vi "Create_filter_points_Sub.vi"(1 "Numeric Value?":bool[](array[boolean]), 4 "No of filter options":i32=100, 5 "Precision":string, 6 "Tolerance":dbl=1.0 format="%.2f", 7 "Bin Matches in":bool[][](array[boolean]), 8 "Numeric Array":dbl[](array[numeric]) format="%.2f", 9 "Bin Names In":string[](array[string]), 10 "String Array":string[](array[string])) -> (2 "Bin Matches":bool[][](array[boolean]), 3 "Bin Names":string[](array[string]))   [LabVIEW 2021]
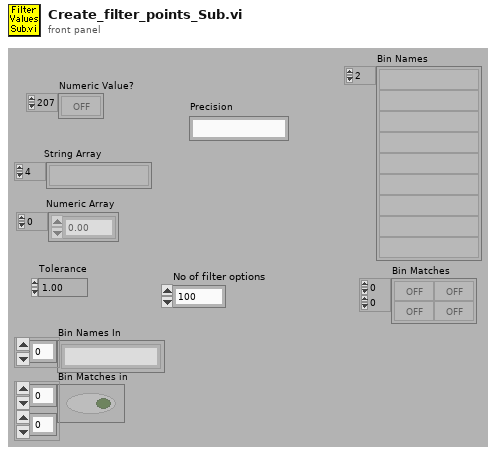
[diagram p1: front panel]
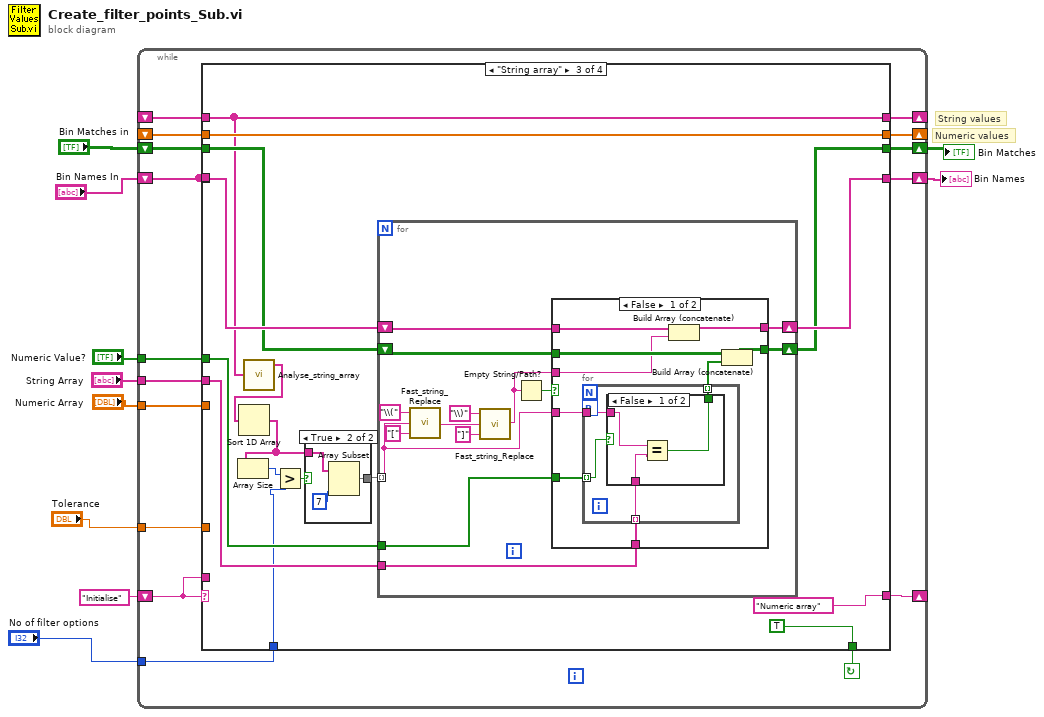
[diagram p0: block diagram]
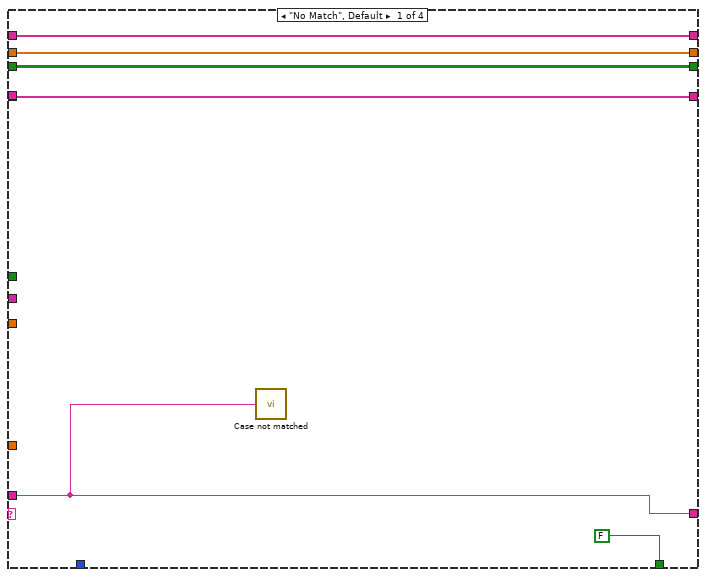
[diagram p2: hidden frame]
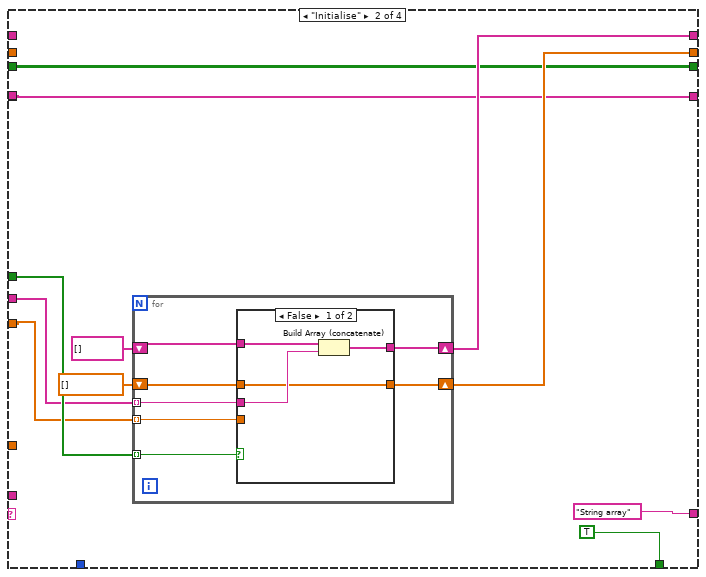
[diagram p3: hidden frame]
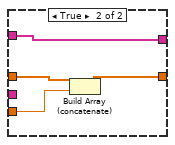
[diagram p4: hidden frame]
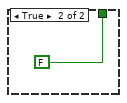
[diagram p6: hidden frame]
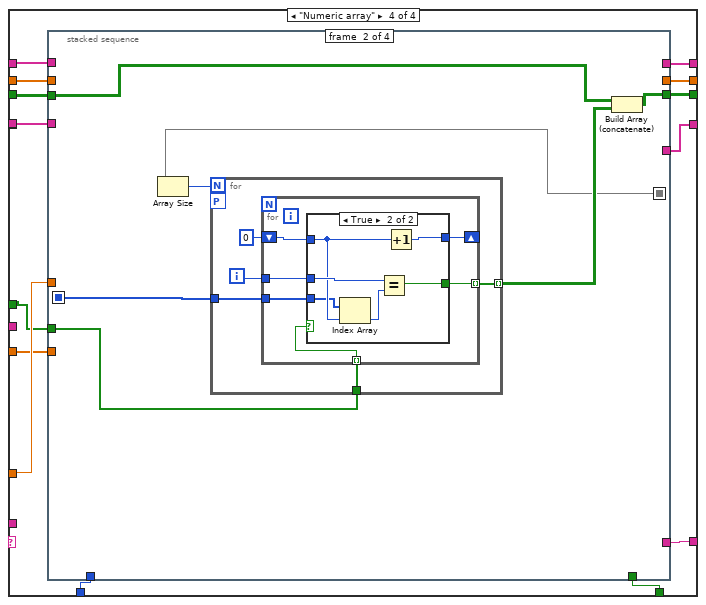
[diagram p8: hidden frame]
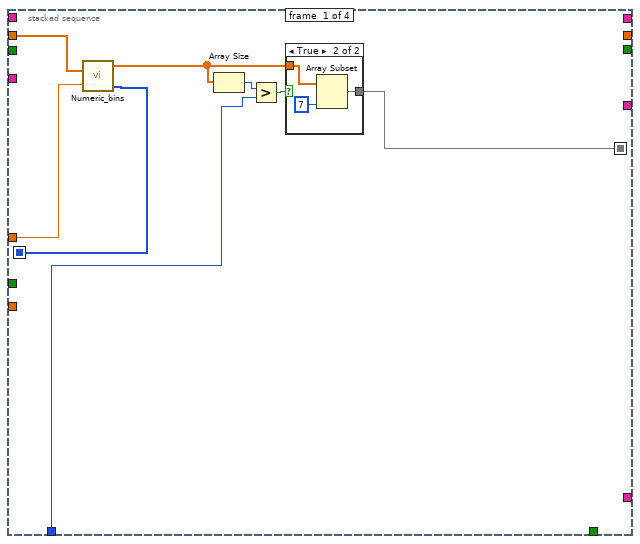
[diagram p9: hidden frame]
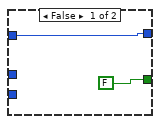
[diagram p11: hidden frame]
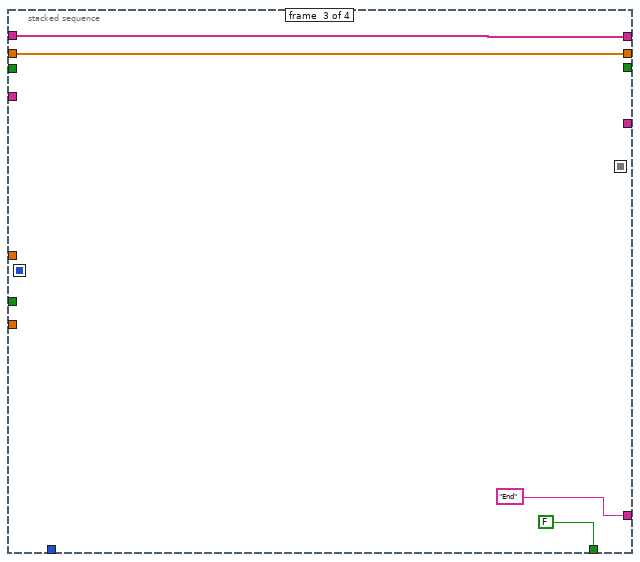
[diagram p12: hidden frame]
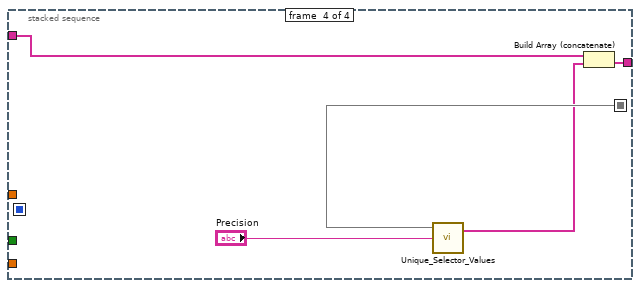
[diagram p13: hidden frame]
diagram:
  # "String values"
  # "Numeric values"
  n1 = while {
    tunnel: "Numeric Value?" -> [w14]
    shift-left: _ -> [w16]
    shift-right: [w15] -> _
    shift-left: "Bin Names In" -> [w17]
    shift-right: [w18] -> w9
    tunnel: "Tolerance" -> [w19]
    shift-left: "Bin Matches in" -> [w23]
    shift-right: [w22] -> w7
    shift-left: _ -> [w20]
    shift-right: [w26] -> _
    shift-left: "Initialise" -> [w21]
    shift-right: [w25] -> _
    tunnel: "Numeric Array" -> [w13]
    tunnel: "String Array" -> [w12]
    tunnel: "No of filter options" -> [w11]
    stop <- w24 continue-if-true
    n2 = case shown="\"String array\"" w21 {
      tunnel: [w31 w35 w73 w121] -> w26
      tunnel: [w27 "String array" "Numeric array" w124] -> w25
      tunnel: [FALSE TRUE TRUE w125] -> w24
      tunnel: w23 -> [w30 w33 w69 w119]
      tunnel: [w30 w33 w68 w118] -> w22
      tunnel: w21 -> [w27 _ _ _]
      tunnel: w20 -> [w31 _ w73 w120]
      tunnel: w19 -> [_ _ _ w122]
      tunnel: [w29 w34 w70 w123] -> w18
      tunnel: w17 -> [w29 w34 w71 w115]
      tunnel: w17 -> [_ _ _ _]
      tunnel: w16 -> [w28 _ w67 w117]
      tunnel: [w28 w36 w67 w116] -> w15
      tunnel: w14 -> [_ w41 w65 w114]
      tunnel: w13 -> [_ w38 _ w113]
      tunnel: w12 -> [_ w40 w66 _]
      tunnel: w11 -> [_ _ w59 w112]
      frame "No Match", Default {
        n3 = call "Case not matched.vi"("Case Name not Matched"=w27) -> ()
      }
      frame "Initialise" {
        n4 = for {
          tunnel: w41 -> [w50] mode=indexing
          shift-right: [w48] -> w36
          shift-left: string[] [] -> [w49]
          shift-right: [w45] -> w35
          shift-left: dbl[] [] -> [w46]
          tunnel: w40 -> [w47] mode=indexing
          tunnel: w38 -> [w44] mode=indexing
          n5 = case shown="False" w50 {
            tunnel: w49 -> [w54 w55]
            tunnel: [w53 w55] -> w48
            tunnel: w47 -> [w52 _]
            tunnel: w46 -> [w51 w58]
            tunnel: [w51 w57] -> w45
            tunnel: w44 -> [_ w56]
            frame False {
              n6 = Build Array (concatenate)(w54, w52) -> (w53:string[])
            }
            frame True {
              n7 = Build Array (concatenate)(w58, w56) -> (w57:dbl[])
            }
          }
        }
      }
      frame "String array" {
        n8 = call "Analyse_string_array.vi"("String array"=w67) -> ("Unique strings"=w64:string[])  [unwired: 2 out]
        n9 = Sort 1D Array(array=w64) -> (sorted array=w61:string[])
        n10 = Array Size(array=w61) -> (size(s)=w62:i32)
        n11 = Greater?(x=w62, y=w59) -> (0:w63:bool)
        n12 = case shown="True" w63 {
          tunnel: w61 -> [w75 w78]
          tunnel: [w75 w77] -> w60
          frame False {
          }
          frame True {
            n13 = Array Subset(array=w78, length=7) -> (w77:string[])  [unwired: 1 in]
          }
        }
        n14 = for {
          tunnel: w66 -> [w82]
          tunnel: w60 -> [w81] mode=indexing
          shift-right: [w85] -> w70
          shift-left: w71 -> [w86]
          shift-right: [w83] -> w68
          shift-left: w69 -> [w84]
          tunnel: w65 -> [w79]
          n15 = call "Fast_string_Replace.vi"("Replace match with:"="[", "Input String"=w81, "regular expression"="\\(") -> ("Output String"=w88:string)  [unwired: 2 out]
          n16 = call "Fast_string_Replace.vi"("Replace match with:"="]", "Input String"=w88, "regular expression"="\\)") -> ("Output String"=w80:string)  [unwired: 2 out]
          n17 = Empty String/Path?(string/path=w80) -> (empty?=w87:bool)
          n18 = case shown="False" w87 {
            tunnel: w86 -> [w101 w111]
            tunnel: [w100 w111] -> w85
            tunnel: w84 -> [w99 w110]
            tunnel: [w98 w110] -> w83
            tunnel: w81 -> [w97 _]
            tunnel: w82 -> [w96 _]
            tunnel: w80 -> [w94 _]
            tunnel: w79 -> [w93 _]
            frame False {
              n19 = for {
                tunnel: w97 -> [w105]
                tunnel: w96 -> [w104] mode=indexing
                tunnel: [w103] -> w95 mode=indexing
                tunnel: w93 -> [w102] mode=indexing
                workers-P: _ -> [_]
                n20 = case shown="False" w102 {
                  tunnel: w105 -> [w108 _]
                  tunnel: w104 -> [w107 _]
                  tunnel: [w106 FALSE] -> w103
                  frame False {
                    n21 = Equal?(x=w108, y=w107) -> (x = y?=w106:bool)
                  }
                  frame True {
                  }
                }
              }
              n22 = Build Array (concatenate)(w101, w94) -> (w100:string[])
              n23 = Build Array (concatenate)(w99, w95) -> (w98:bool[][])
            }
            frame True {
            }
          }
        }
      }
      frame "Numeric array" {
        n24 = stacked-sequence {
          seq-local: [w126 _ _ _] -> [_ w139 _ w170]
          seq-local: [w131 _ _ _] -> [_ w142 _ _]
          tunnel: w122 -> [w132 _ _ _]
          tunnel: [_ _ w164 _] -> w121
          tunnel: w120 -> [w133 _ w164 _]
          tunnel: w119 -> [_ w144 _ _]
          tunnel: [_ w143 _ _] -> w118
          tunnel: [_ _ FALSE _] -> w125
          tunnel: [_ _ "End" _] -> w124
          tunnel: [_ _ _ w172] -> w123
          tunnel: w117 -> [_ _ w165 _]
          tunnel: [_ _ w165 _] -> w116
          tunnel: w115 -> [_ _ _ w171]
          tunnel: w114 -> [_ w141 _ _]
          tunnel: w113 -> [_ _ _ _]
          tunnel: w112 -> [w128 _ _ _]
          frame #0 {
            n25 = call "Numeric_bins.vi"("Values"=w133, "Tolerance"=w132) -> ("Bin Centres"=w127:dbl[], "Bin Index"=w131:i32[])  [unwired: 1 out]
            n26 = Array Size(array=w127) -> (size(s)=w130:i32)
            n27 = Greater?(x=w130, y=w128) -> (0:w129:bool)
            n28 = case shown="True" w129 {
              tunnel: w127 -> [w134 w137]
              tunnel: [w134 w136] -> w126
              frame False {
              }
              frame True {
                n29 = Array Subset(array=w137, length=7) -> (w136:dbl[])  [unwired: 1 in]
              }
            }
          }
          frame #1 {
            n30 = Array Size(array=w139) -> (size(s)=w138:i32)
            n31 = for {
              N: w138 -> [_]
              tunnel: w142 -> [w149]
              tunnel: [w148] -> w140 mode=indexing
              tunnel: w141 -> [w147]
              workers-P: _ -> [_]
              i -> [w145]
              n32 = for {
                tunnel: w149 -> [w151]
                tunnel: w145 -> [w152]
                tunnel: [w150] -> w148 mode=indexing
                tunnel: w147 -> [w155] mode=indexing
                shift-right: [w153] -> _
                shift-left: 0 -> [w154]
                n33 = case shown="True" w155 {
                  tunnel: w154 -> [w157 w161]
                  tunnel: [w157 w163] -> w153
                  tunnel: w152 -> [_ w162]
                  tunnel: w151 -> [_ w160]
                  tunnel: [FALSE w158] -> w150
                  frame False {
                  }
                  frame True {
                    n34 = Index Array(array=w160, index=w161) -> (element=w159:i32)
                    n35 = Equal?(x=w162, y=w159) -> (x = y?=w158:bool)
                    n36 = Increment(x=w161) -> (x+1=w163:i32)
                  }
                }
              }
            }
            n37 = Build Array (concatenate)(w144, w140) -> (w143:bool[][])
          }
          frame #2 {
          }
          frame #3 {
            n38 = call "Unique_Selector_Values.vi"("Precision"="Precision", "Bin Centres"=w170) -> ("Bin Strings"=w168:string[])  [unwired: 1 in, 1 out]
            n39 = Build Array (concatenate)(w171, w168) -> (w172:string[])
          }
        }
      }
    }
  }
  "Bin Names" <- w9
  "Bin Matches" <- w7
